vi "Match Axis NEW (SubVI).vi"(0 "Axis ID":string, 5 "Scale Max, Ga":string(combo), 7 "input string":string, 9 "Visa name in":refnum<visa-resource-name>, 11 "error in":errorcluster) -> (2 "Good\nto read!":bool, 4 "out number":dbl, 6 "Scale Max out":string(combo), 8 "out string":string, 10 "Visa name out":refnum<visa-resource-name>, 13 "status":bool, 15 "error out":errorcluster)   [LabVIEW 2013]
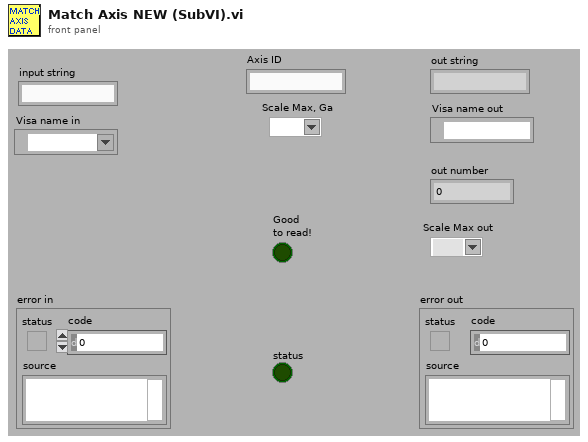
[diagram p1: front panel]
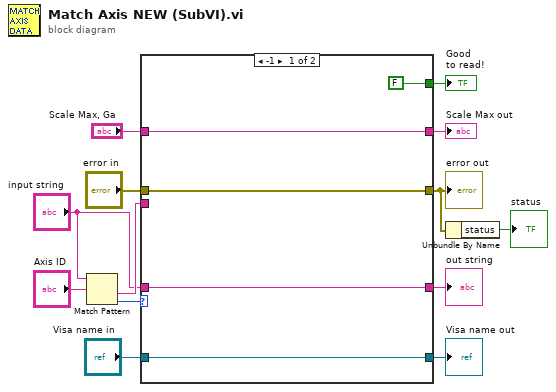
[diagram p0: block diagram]
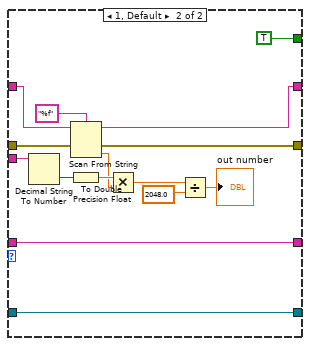
[diagram p2: hidden frame]
diagram:
  n1 = Match Pattern(string="input string", regular expression="Axis ID") -> (after substring=w10:string, offset past match=w9:i32)  [unwired: 3 out]
  n2 = case shown="-1" w9 {
    tunnel: [w18 w29] -> w5
    tunnel: w10 -> [_ w28]
    tunnel: "error in" -> [w18 w27]
    tunnel: "Visa name in" -> [w17 w26]
    tunnel: [w17 w26] -> w13
    tunnel: [w16 w23] -> w7
    tunnel: "Scale Max, Ga" -> [w16 w22]
    tunnel: [w15 w21] -> w2
    tunnel: "input string" -> [w15 w21]
    tunnel: [FALSE ("status") TRUE ("status")] -> w1
    frame -1 {
    }
    frame 1, Default {
      n3 = Decimal String To Number(string=w28) -> (number=w33:i32)  [unwired: 3 out]
      n4 = Scan From String(format string="%f", input string=w22, error in=w27) -> (remaining string=w23:string, error out=w29:errorcluster, output 1=w24:dbl)  [unwired: 1 in, 2 out]
      n5 = To Double Precision Float(number=w33) -> (double precision float=w25:dbl)
      n6 = Multiply(x=w25, y=w24) -> (x*y=w31:dbl)
      n7 = Divide(x=w31, y=2048.0) -> (x/y=→"out number":dbl)
    }
  }
  "Visa name out" <- w13
  "error out" <- w5
  "Scale Max out" <- w7
  "out string" <- w2
  "Good\nto read!" <- w1
  n8 = Unbundle By Name(w5) -> ("status"=→"status":bool)
